vi "dipole_voltage_control(Sub VI).vi"(0 "CH2 Current":dbl=2.2, 1 "CH2 Voltage":dbl=5.0, 2 "CH2 enabled":bool caption="CH2 ON", 3 "CH1 Current":dbl=1.1, 4 "CH1 Voltage":dbl=3.0, 5 "CH1 enabled":bool caption="CH1 ON") -> ()   [LabVIEW 2018]
uses:
  <instrlib>/Rohde&Schwarz HMC 804x Power Supplies/Rohde&Schwarz HMC 804x Power Supplies.lvlib
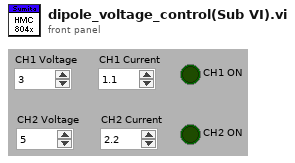
[diagram p1: front panel]
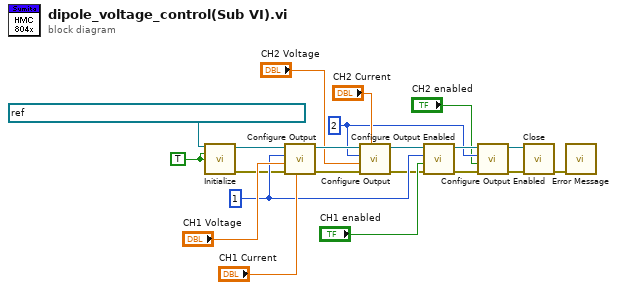
[diagram p0: block diagram]
diagram:
  w9 = TRUE ("ID Query (T: Check)")
  w12 = 2 ("Channel (1)")
  w14 = 1 ("Channel (1)")
  n1 = call <instrlib>:"Initialize.vi"("VISA resource name"=refnum<visa-resource-name> "USB0::0x0AAD::0x0197::5601.1414k02-100769::INSTR", "ID Query (T: Check)"=w9, "Reset (T: Reset)"=w9) -> ("VISA resource name out"=w18:refnum<visa-resource-name>, "error out"=w7:errorcluster)  [unwired: 11 in]
  n2 = call <instrlib>:"Configure Output.vi"("Current (0.0)"="CH1 Current", "error in (no error)"=w7, "Voltage (0.0)"="CH1 Voltage", "Channel (1)"=w14, "VISA resource name"=w18) -> ("error out"=w6:errorcluster, "VISA resource name out"=w17:refnum<visa-resource-name>)  [unwired: 5 in]
  n3 = call <instrlib>:"Configure Output.vi"("Current (0.0)"="CH2 Current", "error in (no error)"=w6, "Voltage (0.0)"="CH2 Voltage", "Channel (1)"=w12, "VISA resource name"=w17) -> ("error out"=w5:errorcluster, "VISA resource name out"=w15:refnum<visa-resource-name>)  [unwired: 5 in]
  n4 = call <instrlib>:"Configure Output Enabled.vi"("error in (no error)"=w5, "Enabled (Off)"="CH1 enabled", "Channel (1)"=w14, "VISA resource name"=w15) -> ("error out"=w4:errorcluster, "VISA resource name out"=w13:refnum<visa-resource-name>)  [unwired: 6 in]
  n5 = call <instrlib>:"Configure Output Enabled.vi"("error in (no error)"=w4, "Enabled (Off)"="CH2 enabled", "Channel (1)"=w12, "VISA resource name"=w13) -> ("error out"=w1:errorcluster, "VISA resource name out"=w2:refnum<visa-resource-name>)  [unwired: 6 in]
  n6 = call <instrlib>:"Close.vi"("error in (no error)"=w1, "VISA resource name"=w2) -> ("error out"=w3:errorcluster)  [unwired: 9 in]
  n7 = call <instrlib>:"Error Message.vi"("error in (no error)"=w3) -> ()  [unwired: 10 in, 5 out]
